vi "poly_control_value_from_name_single.vi"(8 "error in (no error)":errorcluster, 9 "control name":string, 10 "vi ref":refnum<vi>) -> (0 "error out":errorcluster, 1 "Value":variant, 2 "vi ref dup":refnum<vi>, 4 "found?":bool, 5 "ctrl ref":refnum<vi>)   [LabVIEW 2015]
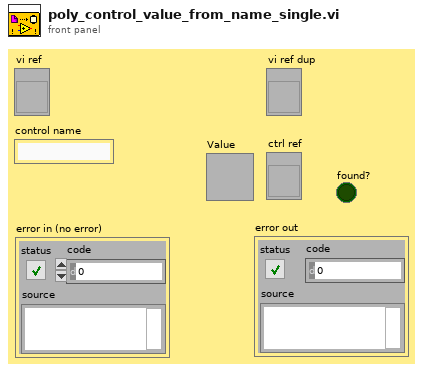
[diagram p1: front panel]
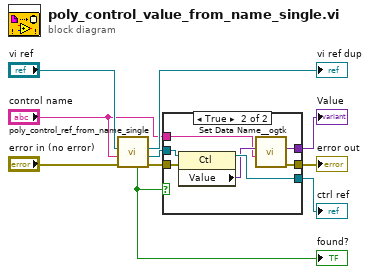
[diagram p0: block diagram]
diagram:
  n1 = call "poly_control_ref_from_name_single.vi"("error in (no error)"="error in (no error)", "control name"="control name", "vi ref"="vi ref") -> ("error out"=w4:errorcluster, "ctrl ref"=w7:refnum<vi>, "vi ref dup"=→"vi ref dup":refnum<vi>, "found?"=w2:bool)  [unwired: 5 in]
  "found?" <- w2
  n2 = case shown="True" w2 {
    tunnel: w7 -> [_ w18]
    tunnel: [_ w17] -> w6
    tunnel: [_ w13] -> w5
    tunnel: w4 -> [w11 w16]
    tunnel: [w11 w15] -> w3
    tunnel: "control name" -> [_ w12]
    frame False {
    }
    frame True {
      n3 = property class="Ctl"(reference=w18, error in=w16) -> (reference out=w17:refnum<vi>, "Value"=w14:variant)  [unwired: 1 out]
      n4 = call <userlib>:"Set Data Name__ogtk.vi"("Data Name"=w12, "Data"=w14) -> ("error out"=w15:errorcluster, "Renamed Data"=w13:variant)  [unwired: 8 in]
    }
  }
  "ctrl ref" <- w6
  "error out" <- w3
  "Value" <- w5
